vi "Configure Synchronize Source.vi"(8 "error in (no error)":errorcluster, 9 "Synchronize Source (0:Voltage)":i32(ring) items=["Voltage", "Current", "Off"], 11 "VISA resource name":refnum<visa-resource-name>) -> (0 "error out":errorcluster, 3 "VISA resource name out":refnum<visa-resource-name>)   [LabVIEW 2019, in "Yokogawa WT300 Series.lvlib"]
doc: "Configures the synchronize source features."
uses:
  Yokogawa WT300 Series.lvlib
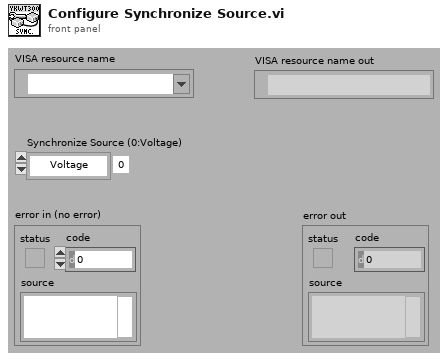
[diagram p1: front panel]
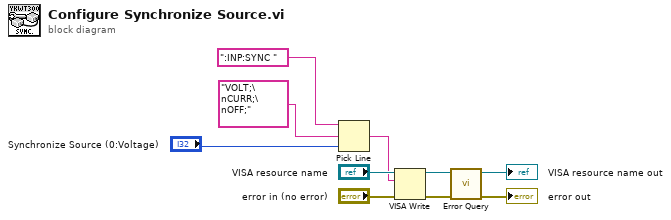
[diagram p0: block diagram]
diagram:
  n1 = Pick Line ("ライン選択")(string ("")=":INP:SYNC ", multi-line string="VOLT;\nCURR;\nOFF;" ("複数行文字列"), line index="Synchronize Source (0:Voltage)") -> (output string=w3:string)
  n2 = VISA Write ("VISA書き込み")(VISA resource name="VISA resource name", write buffer=w3, error in (no error)="error in (no error)") -> (VISA resource name out=w10:refnum<visa-resource-name>, error out=w9:errorcluster)  [unwired: 1 out]
  n3 = call "Error Query.vi"("error in (no error)"=w9, "VISA resource name"=w10) -> ("error out"=→"error out":errorcluster, "VISA resource name out"=→"VISA resource name out":refnum<visa-resource-name>)  [unwired: 6 in, 2 out]
